vi "Ejercicio Array Examen.vi"() -> ()   [LabVIEW 2010]
panel:
  in  "stop":bool
  out "subarray":dbl[](array[numeric])
  out "min index(es)":i32
  out "min value":dbl
  out "max index(es)":i32
  out "max value":dbl
  out "Array":dbl[](array[slide]) scale=0.0..100.0
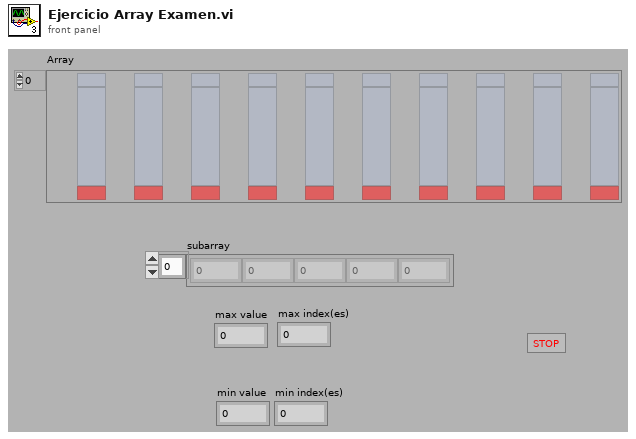
[diagram p1: front panel]
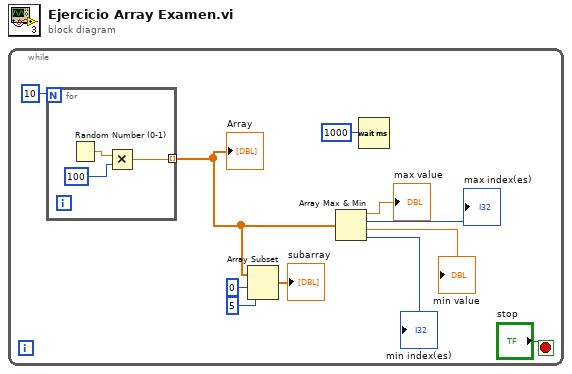
[diagram p0: block diagram]
diagram:
  n1 = while {
    stop <- "stop" stop-if-true
    n2 = for {
      N: 10 -> [_]
      tunnel: [w12] -> w2 mode=indexing
      n3 = Random Number (0-1)() -> (number: 0 to 1=w14:dbl)
      n4 = Multiply(x=w14, y=100) -> (x*y=w12:dbl)
    }
    "Array" <- w2
    n5 = Array Subset(array=w2, index=0, length=5) -> (→"subarray":dbl[])
    n6 = Array Max & Min(array=w2) -> (max value=→"max value":dbl, max index (indices)=→"max index(es)":i32, min value=→"min value":dbl, min index (indices)=→"min index(es)":i32)
    n7 = Wait (ms)(milliseconds to wait=1000) -> ()  [unwired: 1 out]
  }
